vi "MonitorAlert.vi"(8 "error in (no error)":errorcluster, 9 "STOP":bool, 10 "Str Refnum":refnum<vi>, 11 "Handle":i32) -> (0 "error out":errorcluster)   [LabVIEW 2017]
uses:
  <extravilib>/ChannelInstances/Tag-bool/Write With Abort.vi
  <extravilib>/ChannelInstances/Tag-bool/Read With Abort.vi
  <extravilib>/ChannelInstances/Tag-bool/Instantiate.vi
  <extravilib>/ChannelInstances/Tag-bool/EndpointRead.vi
  <extravilib>/ChannelInstances/Tag-bool/Endpoint.vi
  kernel32.dll
  <extravilib>/ChannelInstances/Tag-bool.lvlib
panel:
  out "Array":u8[](array[numeric])
  out "Return":u8
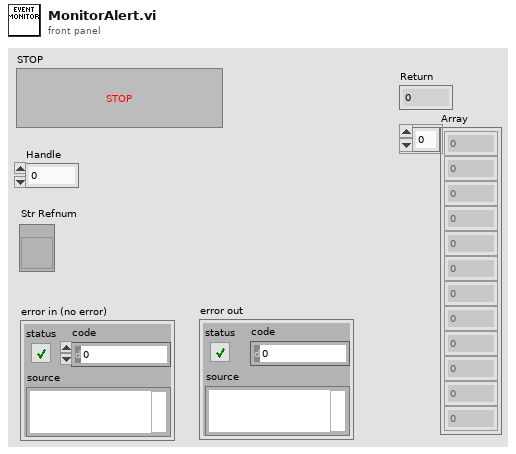
[diagram p1: front panel]
types:
  T1 = typedef "Tag-bool.lvlib/))Channel.ctl" = refnum<queue>
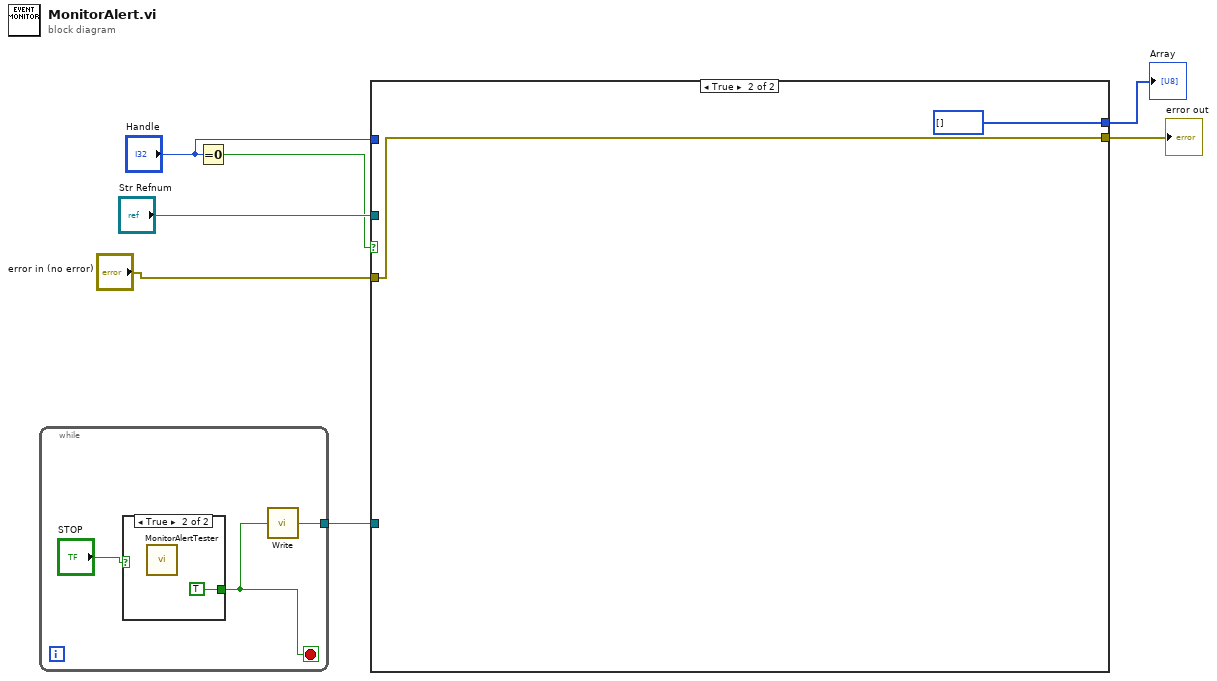
[diagram p0: block diagram]
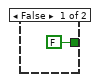
[diagram p2: hidden frame]
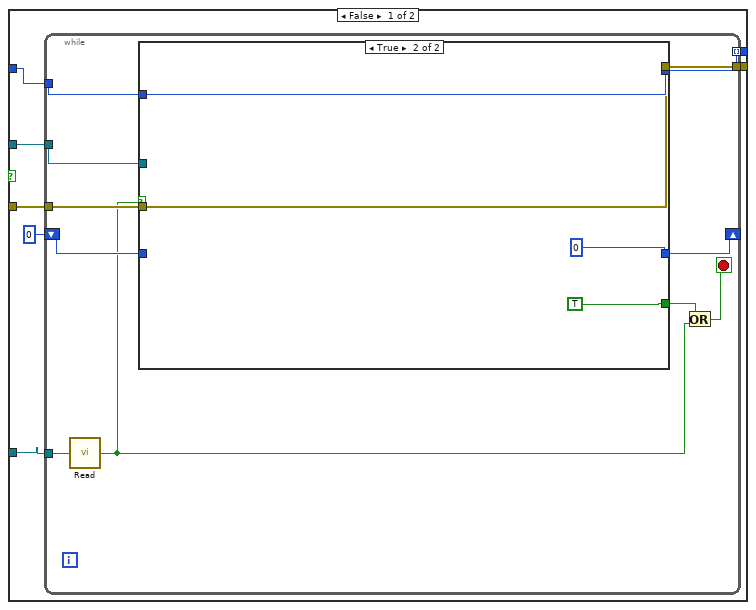
[diagram p3: hidden frame]
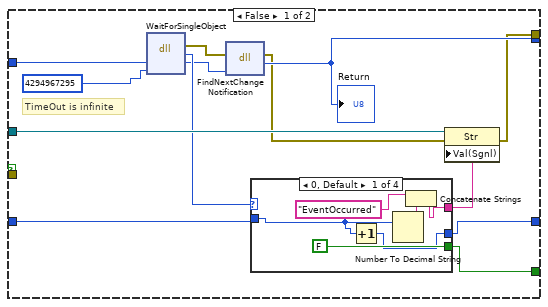
[diagram p4: hidden frame]
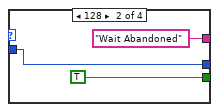
[diagram p5: hidden frame]
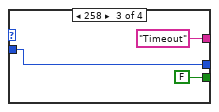
[diagram p6: hidden frame]
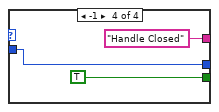
[diagram p7: hidden frame]
diagram:
  n1 = while {
    tunnel: [w10] -> w1
    stop <- w8 stop-if-true
    n2 = case shown="True" "STOP" {
      tunnel: [FALSE TRUE] -> w8
      frame False {
      }
      frame True {
        n3 = call "MonitorAlertTester.vi"() -> ()  [unwired: 12 in]
      }
    }
    n4 = call <extravilib>:"Write.vi"("element"=w8) -> ("channel"=w10:T1)  [unwired: 1 out]
  }
  n5 = Equal To 0?(x="Handle") -> (x = 0?=w4:bool)
  n6 = case shown="True" w4 {
    tunnel: [w19 w64] -> w7
    tunnel: "Str Refnum" -> [w17 _]
    tunnel: "error in (no error)" -> [w16 w64]
    tunnel: "Handle" -> [w15 _]
    tunnel: [w14 u8[] []] -> w2
    tunnel: w1 -> [w13 _]
    frame False {
      n7 = while {
        tunnel: w15 -> [w26]
        tunnel: [w25] -> w19
        shift-right: [w29] -> _
        shift-left: 0 -> [w30]
        tunnel: w17 -> [w28]
        tunnel: w16 -> [w22]
        tunnel: [w27] -> w14 mode=indexing
        tunnel: w13 -> [w21]
        stop <- w23 stop-if-true
        n8 = call <extravilib>:"Read.vi"("channel"=w21) -> ("element"=w20:bool)  [unwired: 1 in, 1 out]
        n9 = case shown="True" w20 {
          tunnel: w30 -> [w43 _]
          tunnel: [w42 0] -> w29
          tunnel: w28 -> [w41 _]
          tunnel: [w40 w61] -> w27
          tunnel: w26 -> [w39 w61]
          tunnel: [w32 w60] -> w25
          tunnel: [w31 TRUE] -> w24
          tunnel: w22 -> [_ w60]
          frame False {
            # "TimeOut is infinite"
            n10 = dll-call lib="kernel32.dll" fn="WaitForSingleObject"("Handle"=w39, "dwMilliseconds"=u32 4294967295) -> (error out=w34:errorcluster, "Return"=w37:u32, "Handle"=w36:i32)  [unwired: 4 in, 1 out]
            n11 = dll-call lib="kernel32.dll" fn="FindNextChangeNotification"(error in=w34, "Handle"=w36) -> (error out=w33:errorcluster, "Return"=w40:u8)  [unwired: 3 in, 1 out]
            "Return" <- w40
            n12 = case shown="0, Default" w37 {
              tunnel: [w46 "Wait Abandoned" ("String") "Timeout" ("String") "Handle Closed" ("String")] -> w35
              tunnel: [FALSE TRUE FALSE TRUE] -> w31
              tunnel: w43 -> [w45 w50 w53 w56]
              tunnel: [w44 w50 w53 w56] -> w42
              frame 0, Default {
                n13 = Increment(x=w45) -> (x+1=w44:i32)
                n14 = Number To Decimal String(number=w45) -> (decimal integer string=w47:string)  [unwired: 1 in]
                n15 = Concatenate Strings("EventOccurred" ("String"), w47) -> (w46:string)
              }
              frame 128 {
              }
              frame 258 {
              }
              frame -1 {
              }
            }
            n16 = property class="Str"(reference=w41, error in=w33, "Val(Sgnl)"=w35) -> (error out=w32:errorcluster)  [unwired: 1 out]
          }
          frame True {
          }
        }
        n17 = Or(x=w24, y=w20) -> (x .or. y?=w23:bool)
      }
    }
    frame True {
    }
  }
  "error out" <- w7
  "Array" <- w2
